vi "Register for Broadcast Events.vi"(8 "error in (no error)":errorcluster, 10 "Event Registration Refnum In":refnum<event-registration>, 11 "Process In":refnum<class "Process.lvclass">) -> (0 "error out":errorcluster, 2 "Event Registration Refnum Out":refnum<event-registration>, 3 "Process Out":refnum<class "Process.lvclass">)   [LabVIEW 2020, in "Process.lvclass"]
doc: "Returns a registration to broadcase messages from the process and any owned processes."
uses:
  Process.lvclass
  Protected/Broadcasting/Broadcast Message Cluster.ctl
  Lifecycle/Lifecycle State.ctl
  Process.lvclass/Process.ctl
  <vilib>/Utility/error.llb/Clear Errors.vi
  <vilib>/Utility/error.llb/Error Cluster From Error Code.vi
  <vilib>/ErrorRing/Error Ring.xnode
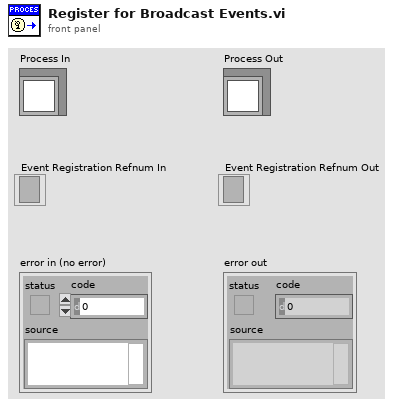
[diagram p1: front panel]
types:
  T1 = typedef "Process.lvclass/Lifecycle State.ctl" = enum16{"Uninitialized", "Initialized", "Started", "Running", "Stopped", "Finished"}
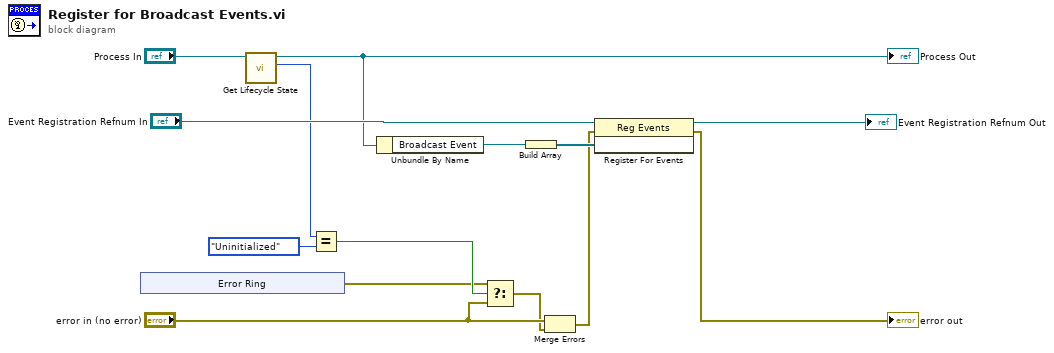
[diagram p0: block diagram]
diagram:
  n1 = xnode "Error Ring"() -> ("error out"=w4:errorcluster)
  n2 = call "Get Lifecycle State.vi"("Process In"="Process In") -> ("Lifecycle State"=w7:T1, "Process Out"=w8:refnum<class "Process.lvclass">)  [unwired: 7 in, 2 out]
  "Process Out" <- w8
  n3 = Equal?(x=w7, y=Lifecycle_State."Uninitialized") -> (x = y?=w5:bool)
  n4 = Unbundle By Name(w8) -> ("Broadcast Event"=w13:refnum<user-event>)
  n5 = Select(t=w4, s=w5, f="error in (no error)") -> (s? t:f=w1:errorcluster)
  n6 = Build Array(w13) -> (w10:refnum<user-event>[])
  n7 = Merge Errors("error in (no error)", w1) -> (w2:errorcluster)
  n8 = register-events(reference="Event Registration Refnum In", error in=w2, w10) -> (reference out=→"Event Registration Refnum Out":refnum<event-registration>, error out=→"error out":errorcluster)
